vi "Replace_Connected_Tracks-2.vi"(5 "Dot Stat Matrix IN":i16[][](array[numeric]), 6 "error IN":errorcluster, 7 "Start Pos IN":i32[](array[numeric]), 8 "Track ID IN":u16[](array[numeric]), 9 "Tracks(PR) IN":dbl[][](array[numeric])) -> (0 "error OUT":errorcluster, 1 "Start Pos OUT":i32[](array[numeric]), 2 "Track ID OUT":u16[](array[numeric]), 3 "Tracks(PR) OUT":dbl[][](array[numeric]), 4 "Dot Status OUT":i16[][](array[numeric]))   [LabVIEW 2017]
doc: "The subVI makes a groups of tracks with same ID (connected)"
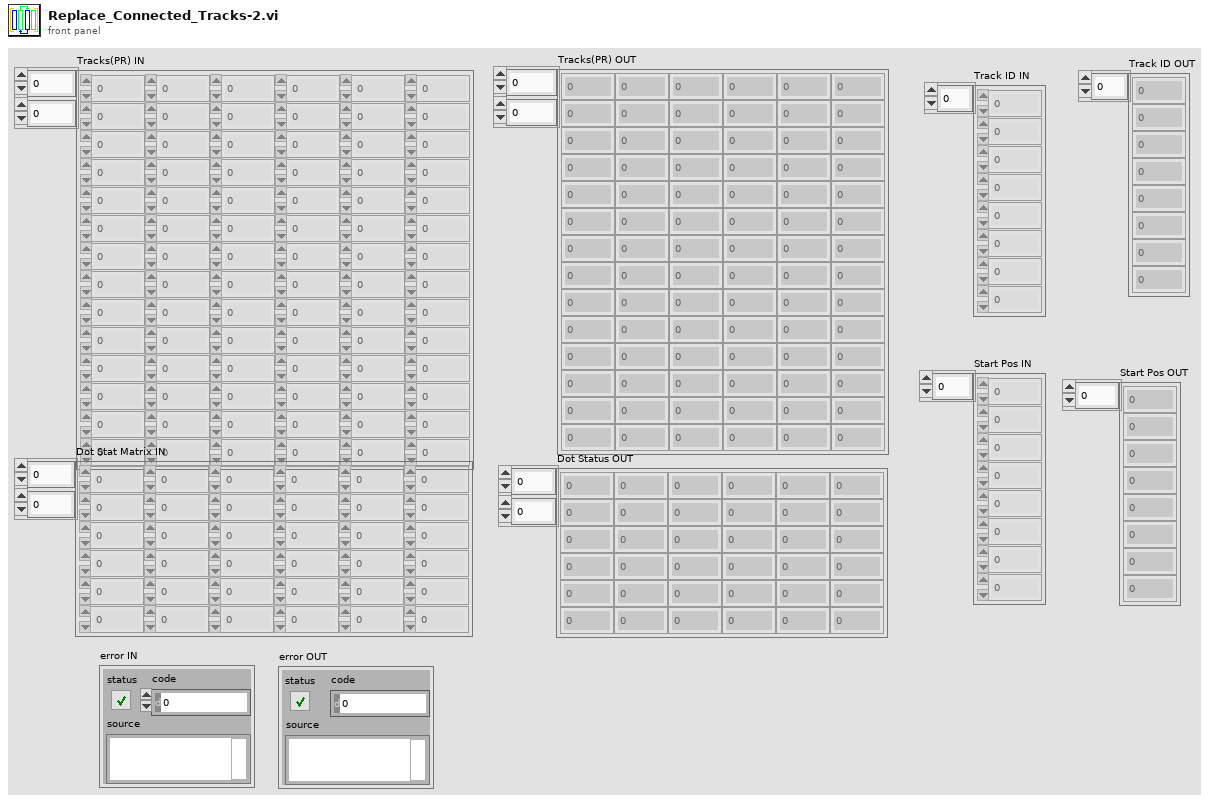
[diagram p1: front panel]
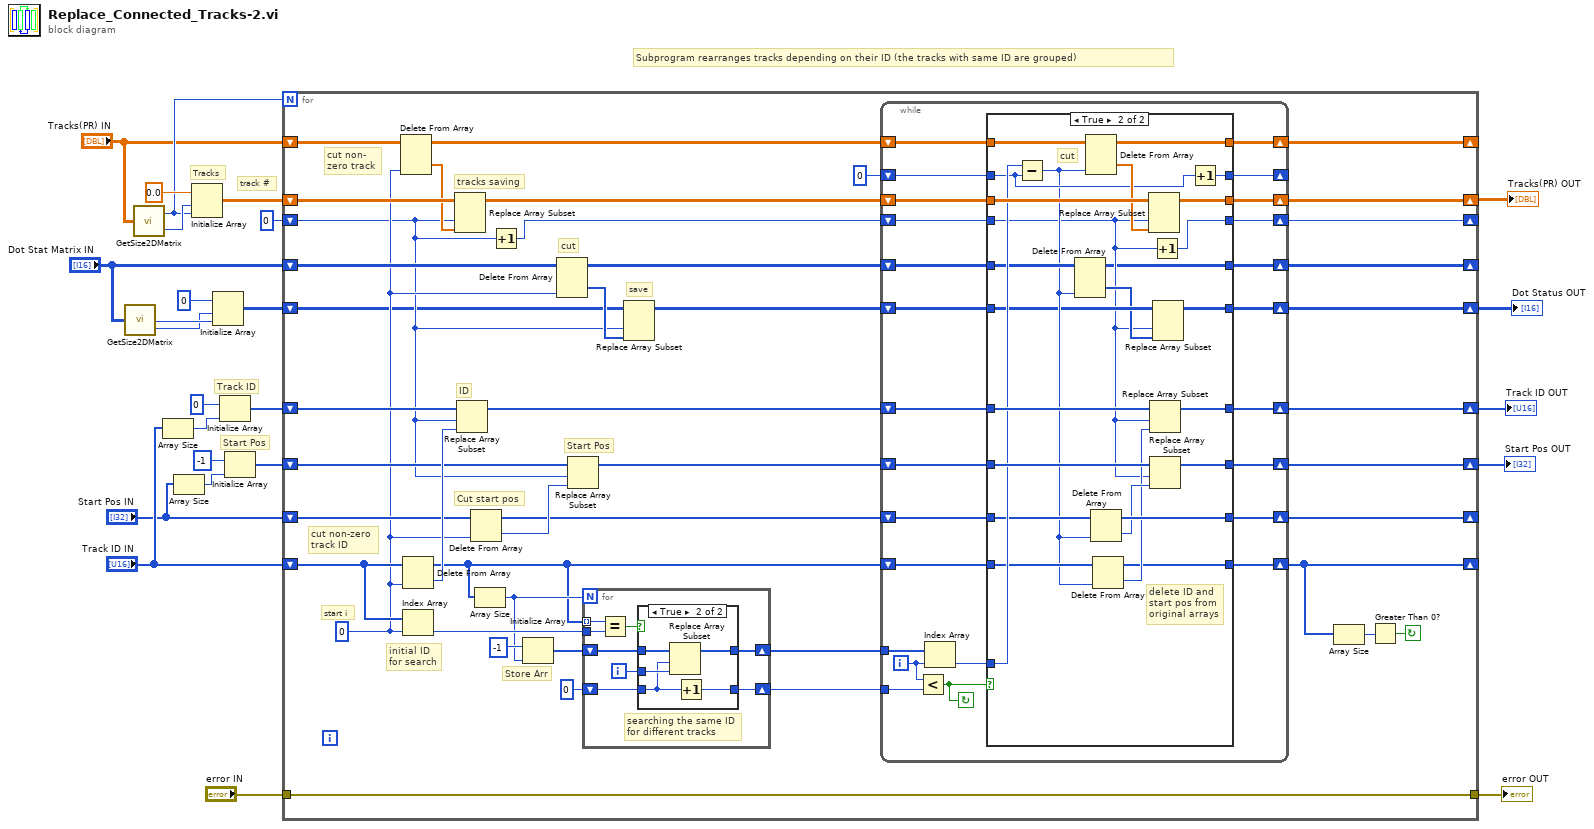
[diagram p0: block diagram]
diagram:
  # "Subprogram rearranges tracks depending on their ID (the tracks with same ID are grouped)"
  # "Start Pos"
  # "track #"
  # "Track ID"
  # "Tracks"
  n1 = call "GetSize2DMatrix.vi"("Array IN (2D)"="Dot Stat Matrix IN") -> ("# Cols"=w4:i32, "# Rows"=w3:i32)
  n2 = call "GetSize2DMatrix.vi"("Array IN (2D)"="Tracks(PR) IN") -> ("# Cols"=w22:i32, "# Rows"=w25:i32)
  n3 = Array Size(array="Track ID IN") -> (size(s)=w18:i32)
  n4 = Array Size(array="Start Pos IN") -> (size(s)=w15:i32)
  n5 = Initialize Array(0.0 ("element"), w25, w22) -> (w23:dbl[][])
  n6 = Initialize Array(i16 0 ("element"), w3, w4) -> (w2:i16[][])
  n7 = Initialize Array(u16 0 ("element"), w18) -> (w19:u16[])
  n8 = Initialize Array(-1 ("element"), w15) -> (w13:i32[])
  n9 = for {
    N: w22 -> [_]
    shift-right: [w43] -> w9
    shift-left: w23 -> [w66]
    shift-right: [w35] -> _
    shift-left: "Tracks(PR) IN" -> [w65]
    shift-right: [w36] -> _
    shift-left: "Track ID IN" -> [w67]
    shift-right: [w45] -> w12
    shift-left: w19 -> [w59]
    shift-right: [w44] -> _
    shift-left: 0 -> [w30]
    shift-right: [w37] -> _
    shift-left: "Start Pos IN" -> [w52]
    shift-right: [w46] -> w11
    shift-left: w13 -> [w51]
    tunnel: "error IN" -> [w42]
    tunnel: [w42] -> w7
    shift-right: [w27] -> _
    shift-left: "Dot Stat Matrix IN" -> [w34]
    shift-right: [w26] -> w1
    shift-left: w2 -> [w29]
    stop <- w47 continue-if-true
    w33 = 0
    # "save"
    # "cut"
    # "Cut start pos"
    # "Start Pos"
    # "ID"
    # "tracks saving"
    # "initial ID\nfor search"
    # "cut non-\nzero track"
    # "cut non-zero\ntrack ID"
    # "Store Arr"
    # "start i"
    n10 = Delete From Array(array=w65, index (col)=w33) -> (deleted portion=w64:dbl[], array with subset deleted=w40:dbl[][])  [unwired: 2 in]
    n11 = Delete From Array(array=w67, index=w33) -> (deleted portion=w58:u16, array with subset deleted=w41:u16[])  [unwired: 1 in]
    n12 = Index Array(array=w67, index=w33) -> (element=w68:u16)
    n13 = Replace Array Subset(array=w66, new element=w64, index (col)=w30) -> (w56:dbl[][])  [unwired: 1 in]
    n14 = Replace Array Subset(array=w59, new element=w58, index=w30) -> (w57:u16[])
    n15 = Delete From Array(array=w52, index=w33) -> (deleted portion=w50:i32, array with subset deleted=w39:i32[])  [unwired: 1 in]
    n16 = Array Size(array=w41) -> (size(s)=w60:i32)
    n17 = Increment(x=w30) -> (x+1=w53:i32)
    n18 = Initialize Array(-1 ("element"), w60) -> (w62:i32[])
    n19 = Delete From Array(array=w34, index (col)=w33) -> (deleted portion=w32:i16[], array with subset deleted=w31:i16[][])  [unwired: 2 in]
    n20 = Replace Array Subset(array=w51, new element=w50, index=w30) -> (w49:i32[])
    n21 = for {
      N: w60 -> [_]
      shift-right: [w133] -> w55
      shift-left: w62 -> [w135]
      tunnel: w68 -> [w137]
      shift-right: [w132] -> w54
      shift-left: 0 -> [w134]
      tunnel: w41 -> [w131] mode=indexing
      i -> [w130]
      # "searching the same ID\nfor different tracks"
      n22 = Equal?(x=w131, y=w137) -> (x = y?=w136:bool)
      n23 = case shown="True" w136 {
        tunnel: w135 -> [w138 w144]
        tunnel: w134 -> [w139 w140]
        tunnel: w130 -> [_ w143]
        tunnel: [w138 w142] -> w133
        tunnel: [w139 w141] -> w132
        frame False {
        }
        frame True {
          n24 = Replace Array Subset(array=w144, new element=w143, index=w140) -> (w142:i32[])
          n25 = Increment(x=w140) -> (x+1=w141:i32)
        }
      }
    }
    n26 = Replace Array Subset(array=w29, new element=w32, index (col)=w30) -> (w28:i16[][])  [unwired: 1 in]
    n27 = while {
      shift-right: [w84] -> w45
      shift-left: w57 -> [w85]
      shift-right: [w86] -> w43
      shift-left: w56 -> [w88]
      tunnel: w55 -> [w93]
      tunnel: w54 -> [w91]
      shift-right: [w83] -> w44
      shift-left: w53 -> [w87]
      shift-right: [w81] -> w46
      shift-left: w49 -> [w82]
      shift-right: [w75] -> _
      shift-left: 0 -> [w77]
      shift-right: [w74] -> w36
      shift-left: w41 -> [w79]
      shift-right: [w73] -> w37
      shift-left: w39 -> [w80]
      shift-right: [w76] -> w35
      shift-left: w40 -> [w78]
      shift-right: [w71] -> w27
      shift-left: w31 -> [w72]
      shift-right: [w69] -> w26
      shift-left: w28 -> [w70]
      i -> [w92]
      stop <- w90 continue-if-true
      n28 = Less?(x=w92, y=w91) -> (x < y?=w90:bool)
      n29 = Index Array(array=w93, index=w92) -> (element=w89:i32)
      n30 = case shown="True" w90 {
        tunnel: w78 -> [w99 w129]
        tunnel: w89 -> [_ w121]
        tunnel: w88 -> [w103 w128]
        tunnel: w87 -> [w101 w106]
        tunnel: [w103 w127] -> w86
        tunnel: w79 -> [w97 w115]
        tunnel: w85 -> [w102 w126]
        tunnel: [w102 w125] -> w84
        tunnel: [w101 w124] -> w83
        tunnel: w80 -> [w98 w118]
        tunnel: w82 -> [w100 w123]
        tunnel: [w100 w122] -> w81
        tunnel: [w99 w119] -> w76
        tunnel: [w98 w117] -> w73
        tunnel: [w97 w111] -> w74
        tunnel: w77 -> [w96 w113]
        tunnel: [w96 w112] -> w75
        tunnel: w72 -> [w95 w110]
        tunnel: [w95 w104] -> w71
        tunnel: [w94 w105] -> w69
        tunnel: w70 -> [w94 w108]
        frame False {
        }
        frame True {
          # "cut"
          # "delete ID and\nstart pos from\noriginal arrays"
          n31 = Subtract(x=w121, y=w113) -> (x-y=w109:i32)
          n32 = Delete From Array(array=w110, index (col)=w109) -> (deleted portion=w107:i16[], array with subset deleted=w104:i16[][])  [unwired: 2 in]
          n33 = Delete From Array(array=w129, index (col)=w109) -> (deleted portion=w120:dbl[], array with subset deleted=w119:dbl[][])  [unwired: 2 in]
          n34 = Delete From Array(array=w118, index=w109) -> (deleted portion=w116:i32, array with subset deleted=w117:i32[])  [unwired: 1 in]
          n35 = Delete From Array(array=w115, index=w109) -> (deleted portion=w114:u16, array with subset deleted=w111:u16[])  [unwired: 1 in]
          n36 = Replace Array Subset(array=w128, new element=w120, index (col)=w106) -> (w127:dbl[][])  [unwired: 1 in]
          n37 = Replace Array Subset(array=w126, new element=w114, index=w106) -> (w125:u16[])
          n38 = Replace Array Subset(array=w123, new element=w116, index=w106) -> (w122:i32[])
          n39 = Increment(x=w106) -> (x+1=w124:i32)
          n40 = Replace Array Subset(array=w108, new element=w107, index (col)=w106) -> (w105:i16[][])  [unwired: 1 in]
          n41 = Increment(x=w113) -> (x+1=w112:i32)
        }
      }
    }
    n42 = Array Size(array=w36) -> (size(s)=w48:i32)
    n43 = Greater Than 0?(x=w48) -> (x > 0?=w47:bool)
  }
  "Tracks(PR) OUT" <- w9
  "Track ID OUT" <- w12
  "Start Pos OUT" <- w11
  "error OUT" <- w7
  "Dot Status OUT" <- w1
